vi "ODE Solver.vi"   [LabVIEW 2014, in "NI_Gmath.lvlib"]
doc: "Solves ordinary differential equations with initial conditions of the following form: X'=F(X,t). You must manually select the polymorphic instance to use."
uses:
  NI_Gmath.lvlib
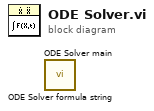
[diagram p0: block diagram]
diagram:
  n1 = call "ODE Solver formula string.vi"() -> ()  [unwired: 9 in, 3 out]
  n2 = call "ODE Solver main.vi"() -> ()  [unwired: 9 in, 3 out]
